vi "generate_2_a.vi"() -> ()   [LabVIEW 2023]
uses:
  <vilib>/Utility/error.llb/DialogType.ctl
  global_vars.vi
panel:
  in  "stop":bool
  out "error out":errorcluster
  in  "error in":errorcluster
  out "Data":i32
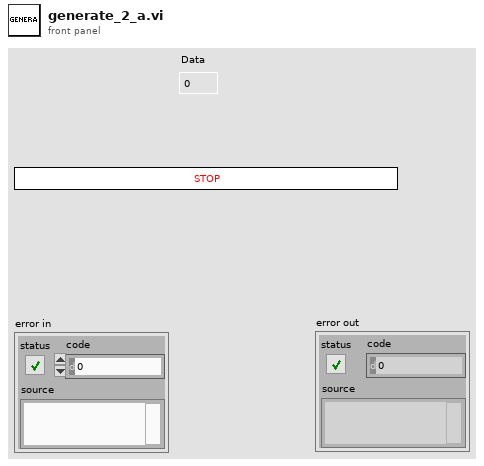
[diagram p1: front panel]
types:
  T1 = typedef "DialogType.ctl" = u16
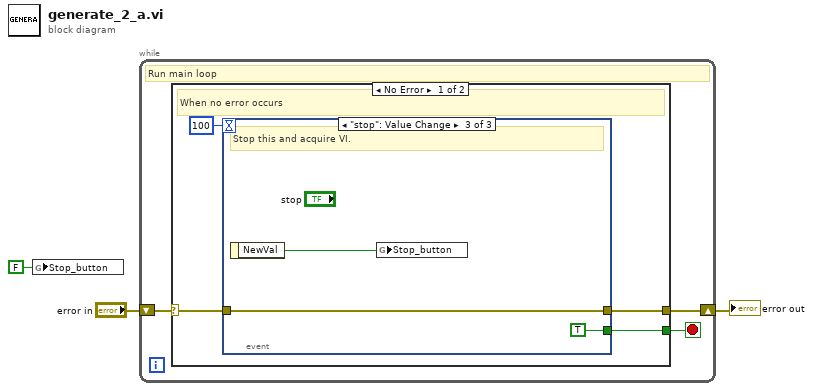
[diagram p0: block diagram]
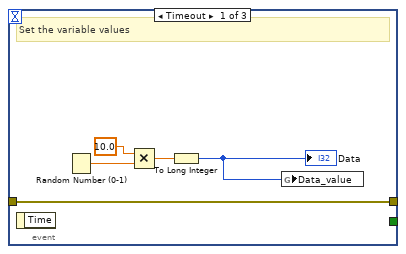
[diagram p2: hidden frame]
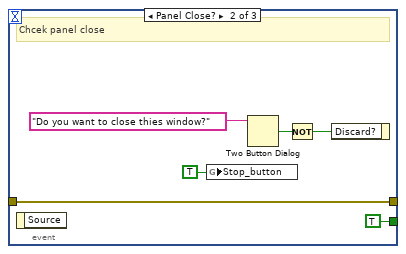
[diagram p3: hidden frame]
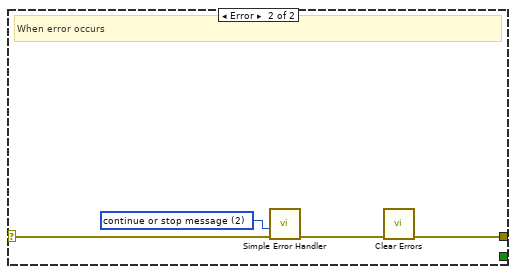
[diagram p4: hidden frame]
diagram:
  n1 = global write "global_vars.vi" "Stop_button"(FALSE ("Stop_button")) -> ()
  n2 = while {
    shift-right: [w5] -> w2
    shift-left: "error in" -> [w6]
    stop <- w4 stop-if-true
    # "Run main loop"
    n3 = case shown="No Error" w6 {
      selector: w6 -> [w9 w28]
      tunnel: [w8 w26] -> w5
      tunnel: [w7 _] -> w4
      frame No Error {
        # "When no error occurs"
        n4 = event shown="[2] \"stop\": Value Change" {
          selector: _ -> [_ _ _]
          dyn-events: _ -> [_ _ _]
          timeout: 100 -> [_ _ _]
          tunnel: [w12 w18 w24] -> w8
          tunnel: w9 -> [w12 w18 w24]
          tunnel: [_ TRUE TRUE] -> w7
          event Timeout {
            # "Set the variable values"
            n5 = event-data() -> ()  [unwired: 1 in, 1 out]
            n6 = Random Number (0-1)() -> (number: 0 to 1=w15:dbl)
            n7 = Multiply(x=10.0, y=w15) -> (x*y=w13:dbl)
            n8 = To Long Integer(number=w13) -> (32bit integer=w11:i32)
            "Data" <- w11
            n9 = global write "global_vars.vi" "Data_value"(w11) -> ()
          }
          event Panel Close? {
            # "Chcek panel close"
            n10 = event-data() -> ()  [unwired: 1 in, 1 out]
            n11 = global write "global_vars.vi" "Stop_button"(TRUE ("Stop_button")) -> ()
            n12 = Two Button Dialog(message="Do you want to close thies window?") -> (T button?=w20:bool)  [unwired: 2 in]
            n13 = Not(x=w20) -> (.not. x?=w19:bool)
            n14 = event-data("Discard?"=w19) -> ()  [unwired: 1 in, 1 out]
          }
          event "stop": Value Change {
            # "Stop this and acquire VI."
            n15 = event-data() -> ("NewVal"=w22:bool)  [unwired: 1 in]
            n16 = global write "global_vars.vi" "Stop_button"(w22) -> ()
          }
        }
      }
      frame Error {
        w25 = T1 2 items=["no dialog", "OK message", "continue or stop message", "OK message + warnings", "continue/stop + warnings"] ("type of dialog (OK msg:1)")
        # "When error occurs"
        n17 = call <vilib>:"Simple Error Handler.vi"("type of dialog (OK msg:1)"=w25, "error in (no error)"=w28) -> ("error out"=w27:errorcluster)  [unwired: 3 in, 4 out]
        n18 = call <vilib>:"Clear Errors.vi"("error in (no error)"=w27) -> ("error out"=w26:errorcluster)  [unwired: 5 in, 1 out]
      }
    }
  }
  "error out" <- w2
